vi "Arduino_DAC_configure.vi"() -> ()   [LabVIEW 2020]
uses:
  Instrument drivers/Arduino/ctls_and_globals/Arduino tx msg cluster.ctl
panel:
  out "Output":dbl
  out "Status comment":string
  in  "Port":refnum<visa-resource-name>="COM18"
  in  "Address":u8=10
  in  "Vout range":u8(ring)=1 items=["0... 5V", "0... 10V"]
  in  "Channel":u8(ring) items=["All", "1", "2", "3", "4", "5", "6", "7", "8", "9", "10", "11", "12", "13", "14", "15", "16"]
  # "Use this vi to configure the AD5754R DAC output range for each channel.\nThis value is retained in EEPROM and recalled on power-up."
  # "PN 20/01/2014"
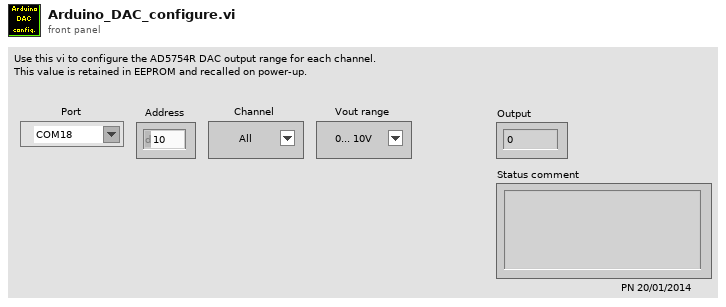
[diagram p1: front panel]
types:
  T1 = typedef "Arduino tx msg cluster.ctl" = cluster{"dest":u8, "A/D/C/I":string, "R/W":string, "chan":u8, "val (float)":sgl}
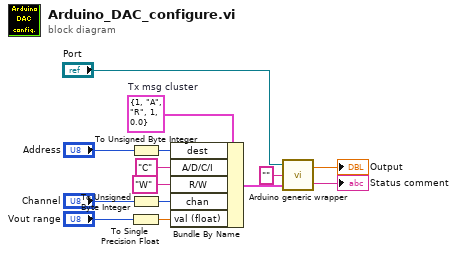
[diagram p0: block diagram]
diagram:
  w8 = T1 {"dest"=1, "A/D/C/I"="A", "R/W"="R", "chan"=1, "val (float)"=0.0}  # Tx msg cluster
  n1 = To Unsigned Byte Integer(number="Address") -> (unsigned 8bit integer=w4:u8)
  n2 = To Unsigned Byte Integer(number="Channel") -> (unsigned 8bit integer=w5:u8)
  n3 = To Single Precision Float(number="Vout range") -> (single precision float=w12:sgl)
  n4 = Bundle By Name(cluster=w8, "dest"=w4, "A/D/C/I"="C" ("A/D"), "R/W"="W", "chan"=w5, "val (float)"=w12) -> (w7:T1)
  n5 = call "Arduino generic wrapper.vi"("Tx msg cluster"=w7, "Channel Name"="", "Port name"="Port") -> ("Scan comment"=→"Status comment":string, "Output"=→"Output":dbl)
